vi "Post-Install Custom Action.vi"(10 "Variant":variant) -> (0 "error out":errorcluster)   [LabVIEW 2020]
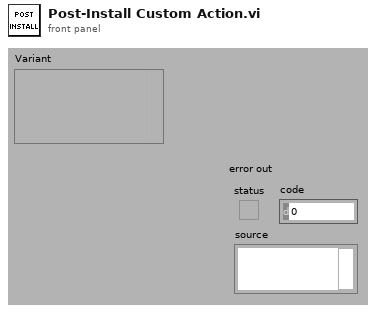
[diagram p1: front panel]
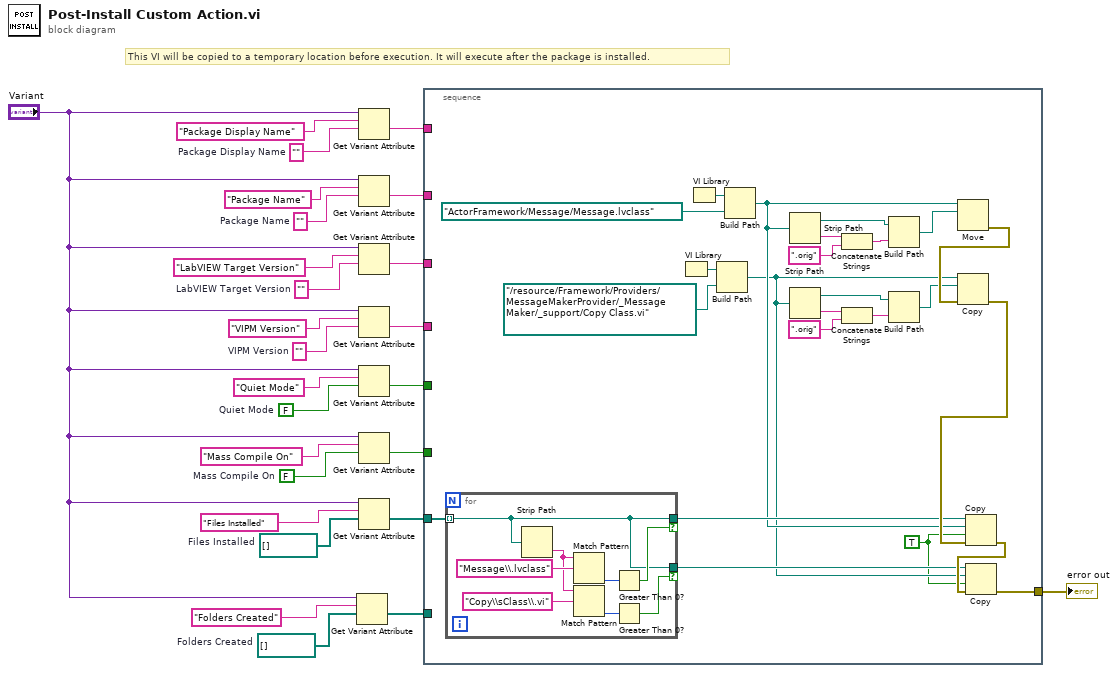
[diagram p0: block diagram]
diagram:
  w2 = path[] []  # Folders Created
  w3 = path[] []  # Files Installed
  w9 = FALSE  # Mass Compile On
  w10 = ""  # Package Display Name
  w17 = FALSE  # Quiet Mode
  w20 = ""  # VIPM Version
  w22 = ""  # LabVIEW Target Version
  w24 = ""  # Package Name
  # "This VI will be copied to a temporary location before execution. It will execute after the package is installed."
  n1 = Get Variant Attribute(Variant="Variant", name="Folders Created", default value (empty Variant)=w2) -> (value=w7:path[])  [unwired: 1 in, 3 out]
  n2 = Get Variant Attribute(Variant="Variant", name="Package Display Name", default value (empty Variant)=w10) -> (value=w16:string)  [unwired: 1 in, 3 out]
  n3 = Get Variant Attribute(Variant="Variant", name="Package Name", default value (empty Variant)=w24) -> (value=w15:string)  [unwired: 1 in, 3 out]
  n4 = Get Variant Attribute(Variant="Variant", name="LabVIEW Target Version", default value (empty Variant)=w22) -> (value=w14:string)  [unwired: 1 in, 3 out]
  n5 = Get Variant Attribute(Variant="Variant", name="VIPM Version", default value (empty Variant)=w20) -> (value=w13:string)  [unwired: 1 in, 3 out]
  n6 = Get Variant Attribute(Variant="Variant", name="Quiet Mode", default value (empty Variant)=w17) -> (value=w12:bool)  [unwired: 1 in, 3 out]
  n7 = Get Variant Attribute(Variant="Variant", name="Mass Compile On", default value (empty Variant)=w9) -> (value=w11:bool)  [unwired: 1 in, 3 out]
  n8 = Get Variant Attribute(Variant="Variant", name="Files Installed", default value (empty Variant)=w3) -> (value=w6:path[])  [unwired: 1 in, 3 out]
  n9 = stacked-sequence {
    tunnel: w16 -> [_]
    tunnel: w15 -> [_]
    tunnel: w14 -> [_]
    tunnel: w13 -> [_]
    tunnel: w12 -> [_]
    tunnel: w11 -> [_]
    tunnel: w6 -> [w47]
    tunnel: w7 -> [_]
    tunnel: [w28] -> w1
    frame #0 {
      w27 = TRUE ("overwrite (F)")
      n10 = for {
        tunnel: w47 -> [w52] mode=indexing
        tunnel: [w52] -> w32 if=w53
        tunnel: [w52] -> w31 if=w51
        n11 = Strip Path(path=w52) -> (name=w56:string)  [unwired: 1 out]
        n12 = Match Pattern(string=w56, regular expression="Message\\.lvclass") -> (offset past match=w55:i32)  [unwired: 1 in, 3 out]
        n13 = Match Pattern(string=w56, regular expression="Copy\\sClass\\.vi") -> (offset past match=w54:i32)  [unwired: 1 in, 3 out]
        n14 = Greater Than 0?(x=w55) -> (x > 0?=w53:bool)
        n15 = Greater Than 0?(x=w54) -> (x > 0?=w51:bool)
      }
      n16 = VI Library() -> (path=w43:path)
      n17 = VI Library() -> (path=w46:path)
      n18 = Build Path(base path=w43, name or relative path=path "../resource/Framework/Providers/MessageMakerProvider/_Message Maker/_support/Copy Class.vi") -> (appended path=w29:path)
      n19 = Build Path(base path=w46, name or relative path=path "ActorFramework/Message/Message.lvclass") -> (appended path=w30:path)
      n20 = Strip Path(path=w30) -> (stripped path=w34:path, name=w42:string)
      n21 = Strip Path(path=w29) -> (stripped path=w35:path, name=w36:string)
      n22 = Concatenate Strings(w42, ".orig" ("string")) -> (w40:string)
      n23 = Concatenate Strings(w36, ".orig" ("string")) -> (w38:string)
      n24 = Build Path(base path=w34, name or relative path=w40) -> (appended path=w39:path)
      n25 = Build Path(base path=w35, name or relative path=w38) -> (appended path=w33:path)
      n26 = Move(source path=w30, 10:w39) -> (error out=w48:errorcluster)  [unwired: 3 in, 2 out]
      n27 = Copy(8:w48, 10:w33, 11:w29) -> (0:w50:errorcluster)  [unwired: 2 in, 2 out]
      n28 = Copy(8:w50, 9:w27, 10:w30, 11:w32) -> (0:w49:errorcluster)  [unwired: 1 in, 2 out]
      n29 = Copy(8:w49, 9:w27, 10:w29, 11:w31) -> (0:w28:errorcluster)  [unwired: 1 in, 2 out]
    }
  }
  "error out" <- w1
